vi "Add Mode Code.vi"(8 "error in":errorcluster, 10 "new Sub Address":refnum<k24>, 11 "Remote Terminal in":refnum<k24>) -> (0 "error out":errorcluster, 3 "Remote Terminal out":refnum<k24>)   [LabVIEW 2020, in "Ballard_1553_Hardware_ni.lvlib"]
uses:
  Ballard_1553_Hardware_ni.lvlib
  C:/Users/Administrator/Desktop/GIT/Ballard-MIL-STD-1553-Custom-Device/Source/System Explorer/SubVIs/Parse XML Ballard/1.2/BTIXML_SerDes.dll
  Ballard-MIL-STD-1553-Custom-Device/Source/System Explorer/SubVIs/Parse XML Ballard/1.2/BTIXML_SerDes.dll
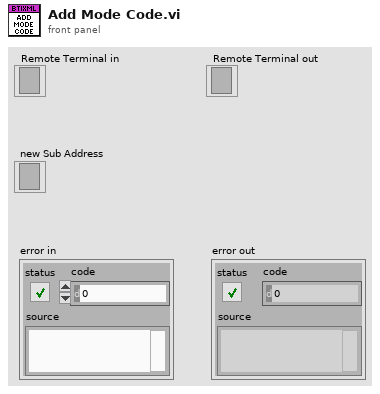
[diagram p1: front panel]
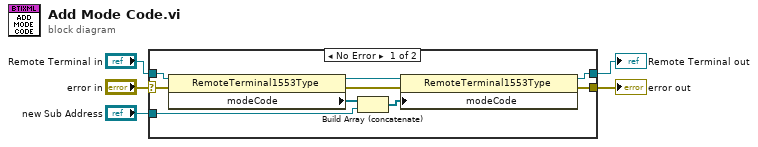
[diagram p0: block diagram]
diagram:
  n1 = case shown="No Error" "error in" {
    selector: "error in" -> [w13 w15]
    tunnel: [w11 w15] -> w5
    tunnel: [w12 w16] -> w1
    tunnel: "Remote Terminal in" -> [w14 w16]
    tunnel: "new Sub Address" -> [w9 _]
    frame No Error {
      n2 = property class="RemoteTerminal1553Type"(reference=w14, error in=w13) -> (reference out=w6:refnum<k24>, error out=w7:errorcluster, "modeCode"=w10:refnum<k24>[])
      n3 = Build Array (concatenate)(w10, w9) -> (w8:refnum<k24>[])
      n4 = property class="RemoteTerminal1553Type"(reference=w6, error in=w7, "modeCode"=w8) -> (reference out=w12:refnum<k24>, error out=w11:errorcluster)
    }
    frame Error {
    }
  }
  "error out" <- w5
  "Remote Terminal out" <- w1
